vi "20170411-lecture3-3 type def studentinfo.vi"() -> ()   [LabVIEW 2014]
uses:
  20170411-lecture3-type def studentinfo.ctl
panel:
  out "student info 3":T1
  in  "student info 2":T1
  in  "student info":T1
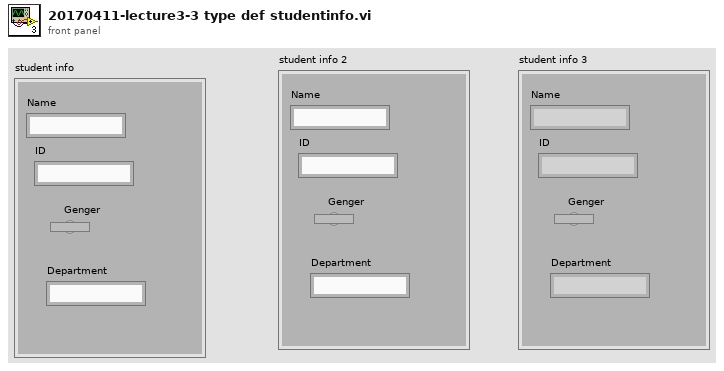
[diagram p1: front panel]
types:
  T1 = typedef "20170411-lecture3-type def studentinfo.ctl" = cluster{"Name":string, "ID":string, "Genger":bool, "Department":string}
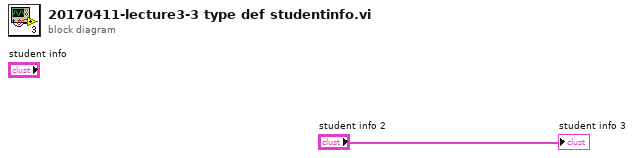
[diagram p0: block diagram]
diagram:
  "student info 3" <- "student info 2"
